vi "SubVi Control.vi"(1 "Boolean":bool, 3 "Boolean 2":bool, 5 "Boolean 3":bool, 7 "Boolean 4":bool, 11 "Boolean 5":bool, 13 "Boolean 6":bool, 15 "Boolean 7":bool, 17 "Boolean 8":bool) -> (23 "Enum":T1)   [LabVIEW 2020]
uses:
  Wash options.ctl
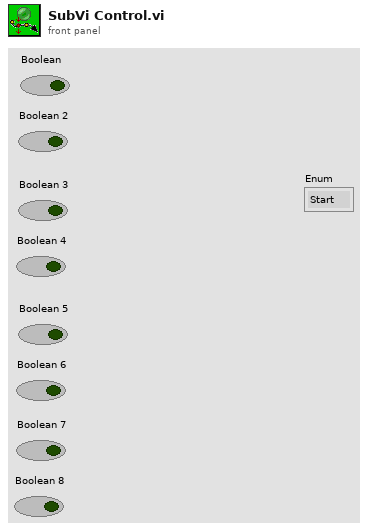
[diagram p1: front panel]
types:
  T1 = typedef "Wash options.ctl" = enum16{"Start", "1", "1.5", "2", "2.3", "2.7", "3", "3.5", "4", "End", "Init"}
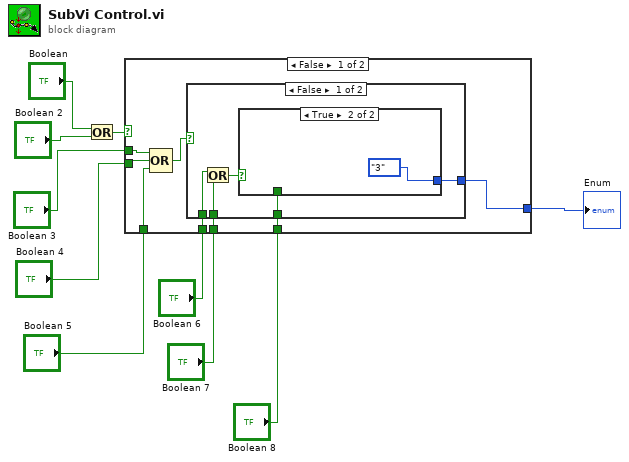
[diagram p0: block diagram]
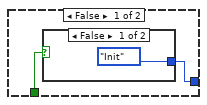
[diagram p2: hidden frame]
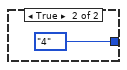
[diagram p3: hidden frame]
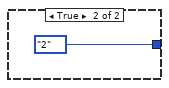
[diagram p4: hidden frame]
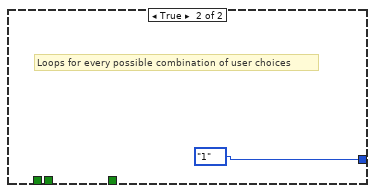
[diagram p5: hidden frame]
diagram:
  n1 = Or(x="Boolean", y="Boolean 2") -> (x .or. y?=w10:bool)
  n2 = case shown="False" w10 {
    tunnel: [w17 Wash_options."1"] -> w1
    tunnel: "Boolean 3" -> [w16 _]
    tunnel: "Boolean 4" -> [w15 _]
    tunnel: "Boolean 5" -> [w14 _]
    tunnel: "Boolean 6" -> [w13 _]
    tunnel: "Boolean 7" -> [w12 _]
    tunnel: "Boolean 8" -> [w11 _]
    frame False {
      n3 = Compound Arithmetic op=OR(w16, w15, w14) -> (w18:bool)
      n4 = case shown="False" w18 {
        tunnel: [w23 Wash_options."2"] -> w17
        tunnel: w13 -> [w21 _]
        tunnel: w12 -> [w20 _]
        tunnel: w11 -> [w19 _]
        frame False {
          n5 = Or(x=w21, y=w20) -> (x .or. y?=w22:bool)
          n6 = case shown="True" w22 {
            tunnel: [w25 Wash_options."3"] -> w23
            tunnel: w19 -> [w24 _]
            frame False {
              n7 = case shown="False" w24 {
                tunnel: [Wash_options."Init" Wash_options."4"] -> w25
                frame False {
                }
                frame True {
                }
              }
            }
            frame True {
            }
          }
        }
        frame True {
        }
      }
    }
    frame True {
      # "Loops for every possible combination of user choices"
    }
  }
  "Enum" <- w1
